vi "Action Runner.vi"(8 "error in (no error)":errorcluster, 9 "Message Data":variant, 10 "Message":string, 11 "Asynchronous Action In":refnum<class "Async Handler.lvclass">) -> (0 "error out":errorcluster, 3 "Asynchronous Action Out":refnum<class "Async Handler.lvclass">)   [LabVIEW 2020, in "Async Handler.lvclass"]
uses:
  Async Handler.lvclass
  Error Handler Interface/Error Handler Interface.lvclass
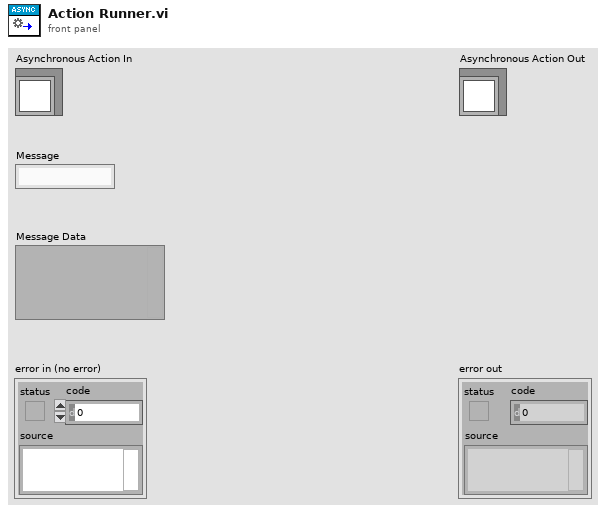
[diagram p1: front panel]
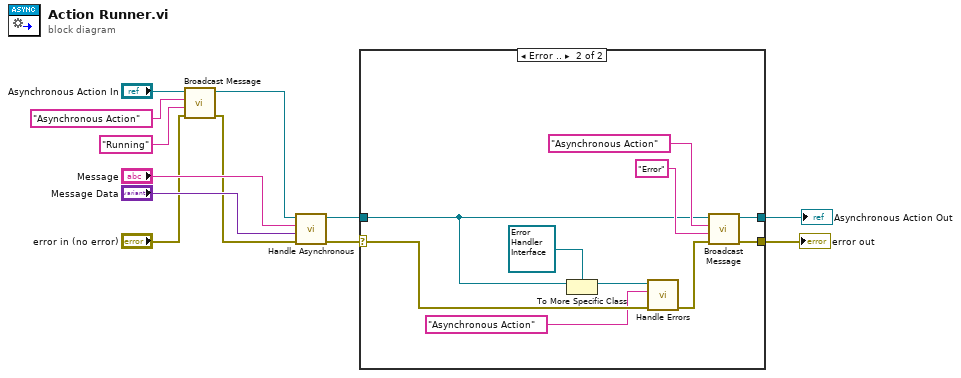
[diagram p0: block diagram]
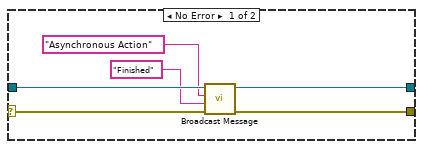
[diagram p2: hidden frame]
diagram:
  n1 = call-dynamic "Broadcast Message.vi"("error in (no error)"="error in (no error)", "Message Data"="Running" ("Message"), "Message"="Asynchronous Action", "Asynchronous Action In"="Asynchronous Action In") -> ("error out"=w3:errorcluster, "Asynchronous Action Out"=w6:refnum<class "Async Handler.lvclass">)  [unwired: 6 in]
  n2 = call-dynamic "Handle Asynchronous.vi"("error in (no error)"=w3, "Message Data"="Message Data", "Message"="Message", "Asynchronous Action In"=w6) -> ("error out"=w7:errorcluster, "Asynchronous Action Out"=w10:refnum<class "Async Handler.lvclass">)  [unwired: 6 in]
  n3 = case shown="Error .." w7 {
    selector: w7 -> [w16 w25]
    tunnel: w10 -> [w17 w20]
    tunnel: [w18 w26] -> w9
    tunnel: [w15 w23] -> w8
    frame No Error {
      n4 = call-dynamic "Broadcast Message.vi"("error in (no error)"=w16, "Message Data"="Finished" ("Message"), "Message"="Asynchronous Action", "Asynchronous Action In"=w17) -> ("error out"=w15:errorcluster, "Asynchronous Action Out"=w18:refnum<class "Async Handler.lvclass">)  [unwired: 6 in]
    }
    frame Error {
      n5 = To More Specific Class(target class=refnum<class "Error Handler Interface.lvclass"> refnum ("Process In"), reference=w20) -> (specific class reference=w19:refnum<class "Error Handler Interface.lvclass">)  [unwired: 1 in, 1 out]
      n6 = call-dynamic "Handle Errors.vi"("error in (no error)"=w25, "Location"="Asynchronous Action" ("format string"), "Error Handler Interface In"=w19) -> ("error out"=w24:errorcluster)  [unwired: 7 in, 1 out]
      n7 = call-dynamic "Broadcast Message.vi"("error in (no error)"=w24, "Message Data"="Error" ("Message"), "Message"="Asynchronous Action", "Asynchronous Action In"=w20) -> ("error out"=w23:errorcluster, "Asynchronous Action Out"=w26:refnum<class "Async Handler.lvclass">)  [unwired: 6 in]
    }
  }
  "error out" <- w8
  "Asynchronous Action Out" <- w9
